vi "Extract Multiple Tone Information N Chan - N Specs.vi"(0 "time signals in":waveform(dbl)[](array[waveform]), 5 "export mode":T1(array[ring]), 7 "threshold":dbl[](array[numeric]) format="%#_6p", 9 "max num tones":i32[](array[numeric]), 11 "error in (no error)":errorcluster, 12 "output sorting":i32(ring) items=["increasing frequency", "decreasing amplitude"]) -> (3 "exported signals":T3(array[cluster]) {"exported spectrum (dB)"."dB Spectrum (Hann)" format="%.2p"; "exported spectrum (dB)"."df" format="%.2p"; "exported spectrum (dB)"."f0" format="%.2p"}, 4 "multiple tone information":T2(array[cluster]) {"multiple tone information"."detected phase (deg)" format="%_6g"; "multiple tone information"."detected amplitude" format="%_6p"; "multiple tone information"."detected frequency" format="%_6p"}, 15 "error out":errorcluster)   [LabVIEW 2020, in "NI_MAPro.lvlib"]
doc: "Returns the frequency, amplitude, and phase for each signal tone whose amplitude exceeds a specified <B>threshold</B>. Wire data to the <B>time signal in</B> input to determine the polymorphic instance to use or manually select the instance."
uses:
  NI_MAPro.lvlib
  NI_MABase.lvlib
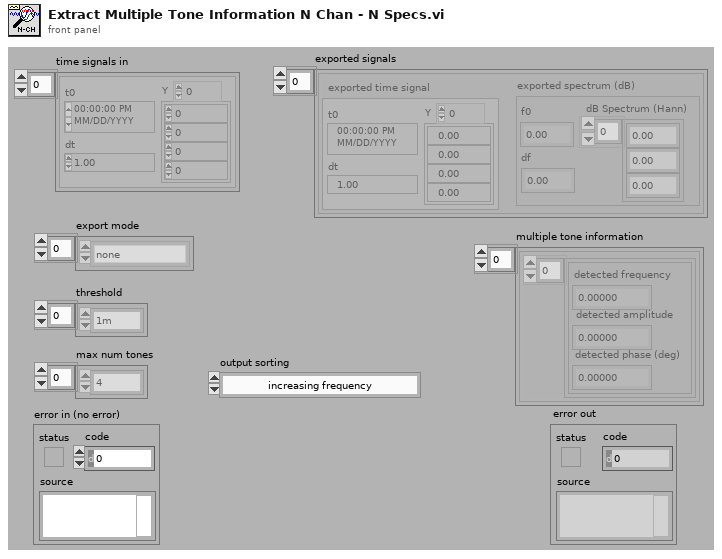
[diagram p1: front panel]
types:
  T1 = enum32{"none", "input signal", "detected signal", "residual signal"}[]
  T2 = cluster{"multiple tone information":cluster{"detected frequency":dbl, "detected amplitude":dbl, "detected phase (deg)":dbl}[]}[]
  T3 = cluster{"exported time signal":waveform(dbl), "exported spectrum (dB)":cluster{"f0":dbl, "df":dbl, "dB Spectrum (Hann)":dbl[]}}[]
  T4 = cluster{"exported time signal":waveform(dbl), "exported spectrum (dB)":cluster{"f0":dbl, "df":dbl, "dB Spectrum (Hann)":dbl[]}}
  T5 = cluster{"detected frequency":dbl, "detected amplitude":dbl, "detected phase (deg)":dbl}[]
  T6 = cluster{"multiple tone information":cluster{"detected frequency":dbl, "detected amplitude":dbl, "detected phase (deg)":dbl}[]}
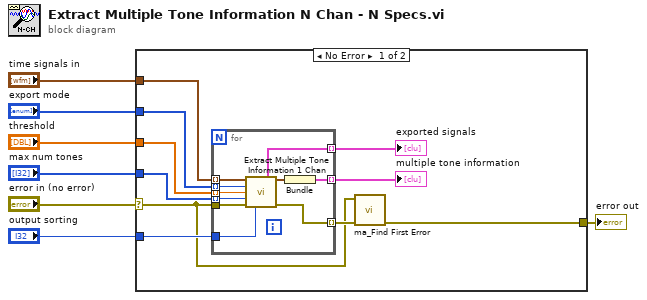
[diagram p0: block diagram]
diagram:
  n1 = case shown="No Error" "error in (no error)" {
    selector: "error in (no error)" -> [w8 w28]
    tunnel: "output sorting" -> [w17 _]
    tunnel: "time signals in" -> [w16 _]
    tunnel: [w12 w28] -> w5
    tunnel: "export mode" -> [w11 _]
    tunnel: "threshold" -> [w10 _]
    tunnel: "max num tones" -> [w9 _]
    frame No Error {
      n2 = for {
        tunnel: w8 -> [w27]
        tunnel: w9 -> [w26] mode=indexing
        tunnel: w10 -> [w25] mode=indexing
        tunnel: w11 -> [w24] mode=indexing
        tunnel: w17 -> [w23]
        tunnel: w16 -> [w22] mode=indexing
        tunnel: [w21] -> w15 mode=indexing
        tunnel: [w19] -> w14 mode=indexing
        tunnel: [w18] -> w13 mode=indexing
        n3 = call "Extract Multiple Tone Information 1 Chan.vi"("time signal in"=w22, "export mode"=w24, "threshold"=w25, "max num tones"=w26, "error in (no error)"=w27, "output sorting"=w23) -> ("exported signals"=w21:T4, "multiple tone information"=w20:T5, "error out"=w18:errorcluster)  [unwired: 7 out]
        n4 = Bundle("multiple tone information"=w20) -> (w19:T6)  [unwired: 1 in]
      }
      "exported signals" <- w15
      "multiple tone information" <- w14
      n5 = call "ma_Find First Error.vi"("error array in"=w13, "error in 1 (no error)"=w8) -> ("error out"=w12:errorcluster)  [unwired: 2 in, 3 out]
    }
    frame Error {
    }
  }
  "error out" <- w5
